vi "Ctor.vi"(4 "Port Config":T1={"Baud (115200)"=115200, "Data Bits (8)"=8, "Stop Bits (1)"=10, "Flow Control"=0, "Use LineTerm?"=FALSE, "LineTerm (\\n)"="\n", "Timeout ms (10000)"=10000, "Parity (None)"=enum."None"} {"Flow Control" items=["None", "XON/XOFF", "RTS/CTS", "XON/XOFF & RTS/CTS", "DTR/DSR", "XON/XOFF & DTR/DSR"]; "Stop Bits (1)" items=["1.0"=10, "1.5"=15, "2.0"=20]}, 8 "error in (no error)":errorcluster, 10 "Command Queue":T5, 11 "VISA resource name":refnum<visa-resource-name>) -> (0 "error out":errorcluster, 3 "Serial Stream out":refnum<class "Serial Stream.lvclass">)   [LabVIEW 2020, in "Stream-Serial.lvlib" / "Serial Stream.lvclass"]
uses:
  Serial Stream.lvclass
  Command Queue.ctl
  Client Command.ctl
  Serial Client/Port Config.ctl
  Serial Client/Stop Bits.ctl
  Serial Client/Flow Control.ctl
  Serial Client/Parity.ctl
  Ref Data.ctl
  Serial Stream.lvclass/Serial Stream.ctl
  Stream-Serial.lvlib
  Serial Client/Serial Client.lvclass
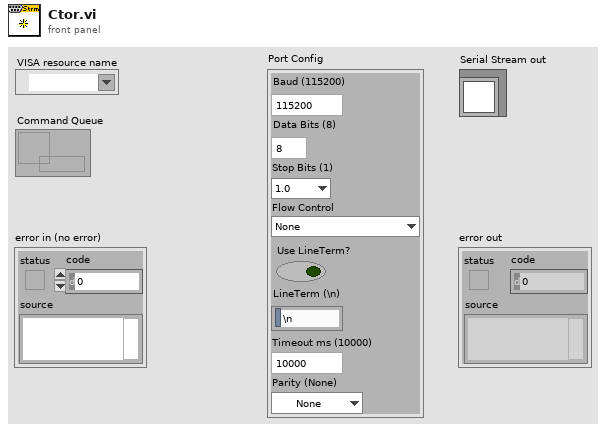
[diagram p1: front panel]
types:
  T1 = typedef "Stream-Serial.lvlib/Serial Client.lvclass/Port Config.ctl" = cluster{"Baud (115200)":u32, "Data Bits (8)":u8, "Stop Bits (1)":T2, "Flow Control":T3, "Use LineTerm?":bool, "LineTerm (\\n)":string, "Timeout ms (10000)":i32, "Parity (None)":T4}
  T2 = typedef "Stream-Serial.lvlib/Serial Client.lvclass/Stop Bits.ctl" = u16
  T3 = typedef "Stream-Serial.lvlib/Serial Client.lvclass/Flow Control.ctl" = u16
  T4 = typedef "Stream-Serial.lvlib/Serial Client.lvclass/Parity.ctl" = enum16{"None", "Odd", "Even", "Mark", "Space"}
  T5 = typedef "Stream-Serial.lvlib/Command Queue.ctl" = refnum<queue>
  T6 = typedef "Stream-Serial.lvlib/Serial Stream.lvclass/Ref Data.ctl" = cluster{"Command Queue":T5}
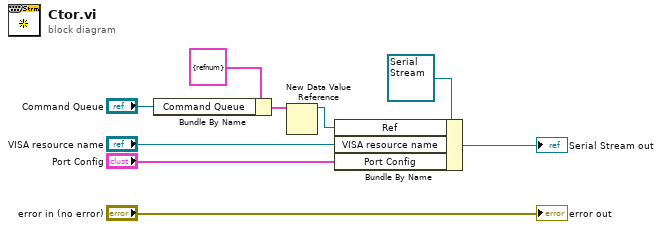
[diagram p0: block diagram]
diagram:
  n1 = Bundle By Name(cluster=T6 {"Command Queue"=refnum} ("Ref Data"), "Command Queue"="Command Queue") -> (w3:T6)
  n2 = New Data Value Reference(data value=w3) -> (data value reference=w2:refnum<data-value>)  [unwired: 1 in, 1 out]
  n3 = Bundle By Name(cluster=refnum<class "Serial Stream.lvclass"> refnum ("Serial Stream in"), "Ref"=w2, "VISA resource name"="VISA resource name", "Port Config"="Port Config") -> (→"Serial Stream out":refnum<class "Serial Stream.lvclass">)
  "error out" <- "error in (no error)"
